vi "Get_AO_Array.vi"(0 "reference in":refnum<class "FPGA_Concrete.lvclass">, 11 "error in (no error)":errorcluster) -> (4 "reference out":refnum<class "FPGA_Concrete.lvclass">, 6 "AOs":dbl[](array[numeric]), 15 "error out":errorcluster)   [LabVIEW 2019, in "FPGA_Concrete.lvclass"]
uses:
  FPGA_Concrete.lvclass
  FPGA_Concrete.lvclass/FPGA_Concrete.ctl
  <vilib>/Utility/error.llb/Error Cluster From Error Code.vi
  <vilib>/rvi/errors/niLvFpgaAdjustHostInterfaceError.vi
  <vilib>/rvi/interface/nirviReadWriteControl/nirviReadWriteControl.xnode
  FPGA VI Reference.ctl
  NiFpgaLv.dll
  <vilib>/rvi/interface/Simulation/niFpgaSimulationCallBeginRW.vi
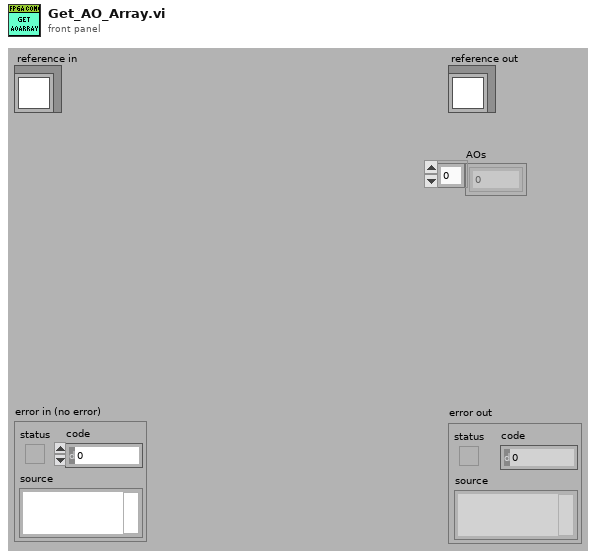
[diagram p1: front panel]
types:
  T1 = typedef "FPGA_Concrete.lvclass/FPGA VI Reference.ctl" = refnum<k20>
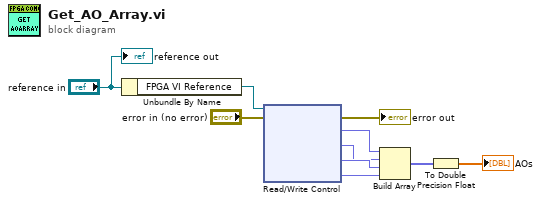
[diagram p0: block diagram]
diagram:
  n1 = Unbundle By Name("reference in") -> ("FPGA VI Reference"=w9:T1)
  n2 = xnode "Read/Write Control"("FPGA VI Reference In"=w9, "error in"="error in (no error)") -> ("error out"=→"error out":errorcluster, "Mod5/AO0"=w3:fxp<+/-,20,5>, "Mod5/AO1"=w4:fxp<+/-,20,5>, "Mod5/AO2"=w5:fxp<+/-,20,5>, "Mod5/AO3"=w6:fxp<+/-,20,5>)  [unwired: 1 out]
  n3 = Build Array(w3, w4, w5, w6) -> (w2:fxp<+/-,20,5>[])
  n4 = To Double Precision Float(number=w2) -> (double precision float=→"AOs":dbl[])
  "reference out" <- "reference in"
